vi "Excel.vi"   [LabVIEW 2020]
panel:
  # "ActiveX Example"
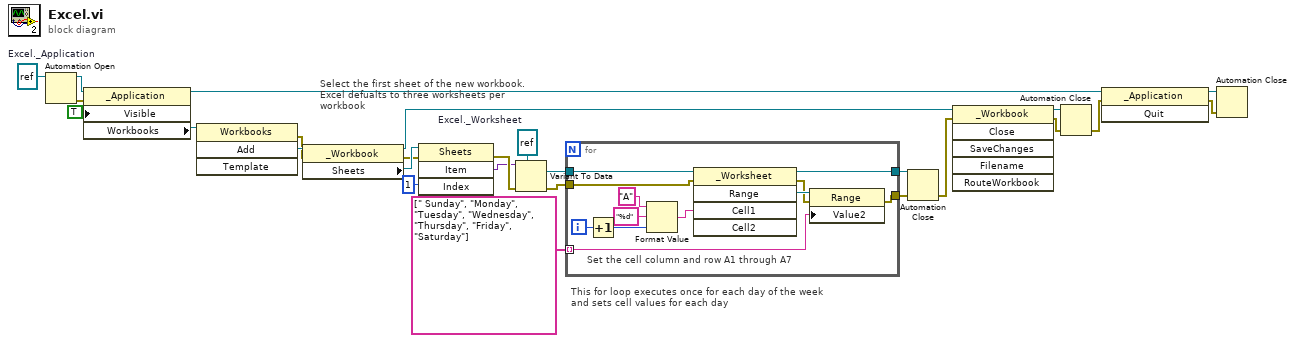
[diagram p0: block diagram]
diagram:
  w19 = refnum<k7> refnum  # Excel._Worksheet
  w26 = refnum<k7> refnum  # Excel._Application
  # "Select the first sheet of the new workbook.  Excel defualts to three worksheets per workbook"
  # "This for loop executes once for each day of the week and sets cell values for each day"
  n1 = Automation Open(Automation Refnum=w26) -> (Automation Refnum=w16:refnum<k7>, error out=w13:errorcluster)  [unwired: 3 in]
  n2 = property class="_Application"(reference=w16, error in=w13, "Visible"=TRUE) -> (reference out=w1:refnum<k7>, "Workbooks"=w2:refnum<k7>)  [unwired: 1 out]
  n3 = invoke class="Workbooks" method="Add"(reference=w2) -> (error out=w10:errorcluster, "Add"=w14:refnum<k7>)  [unwired: 3 in, 2 out]
  n4 = property class="_Workbook"(reference=w14, error in=w10) -> (reference out=w7:refnum<k7>, error out=w21:errorcluster, "Sheets"=w22:refnum<k7>)
  n5 = invoke class="Sheets" method="Item"(reference=w22, error in=w21, "Index"=1) -> (error out=w18:errorcluster, "Item"=w17:variant)  [unwired: 1 in, 2 out]
  n6 = Variant To Data(error in=w18, type=w19, Variant=w17) -> (data=w24:refnum<k7>, error out=w25:errorcluster)
  n7 = for {
    tunnel: string[] [" Sunday", "Monday", "Tuesday", "Wednesday", "Thursday", "Friday", "Saturday"] -> [w31] mode=indexing
    tunnel: w24 -> [w30]
    tunnel: w25 -> [w29]
    tunnel: [w28] -> w12
    tunnel: [w27] -> w11
    i -> [w33]
    # "Set the cell column and row A1 through A7"
    n8 = Increment(x=w33) -> (x+1=w36:i32)
    n9 = Format Value(string ("")="A", format string="%d", value (0)=w36) -> (output string=w32:string)
    n10 = invoke class="_Worksheet" method="Range"(reference=w30, error in=w29, "Cell1"=w32) -> (reference out=w28:refnum<k7>, error out=w37:errorcluster, "Range"=w38:refnum<k7>)  [unwired: 2 in, 2 out]
    n11 = property class="Range"(reference=w38, error in=w37, "Value2"=w31) -> (error out=w27:errorcluster)  [unwired: 1 out]
  }
  n12 = Automation Close(3:w11, 5:w12) -> (0:w5:errorcluster)
  n13 = invoke class="_Workbook" method="Close"(reference=w7, error in=w5) -> (reference out=w9:refnum<k7>, error out=w8:errorcluster)  [unwired: 4 in, 4 out]
  n14 = Automation Close(3:w8, 5:w9) -> (0:w6:errorcluster)
  n15 = invoke class="_Application" method="Quit"(reference=w1, error in=w6) -> (reference out=w3:refnum<k7>, error out=w4:errorcluster)  [unwired: 1 in, 1 out]
  n16 = Automation Close(3:w4, 5:w3) -> ()  [unwired: 1 out]
